vi "Heading string.vi"() -> ()   [LabVIEW 2011]
panel:
  out "String":string
  in  "Array":string[](array[string])
  out "Heading string":string
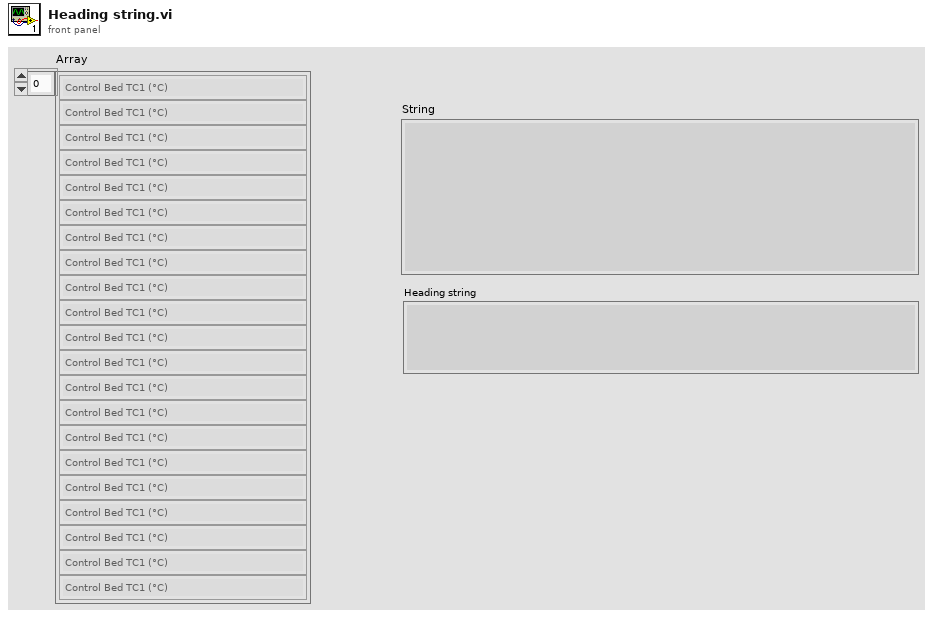
[diagram p1: front panel]
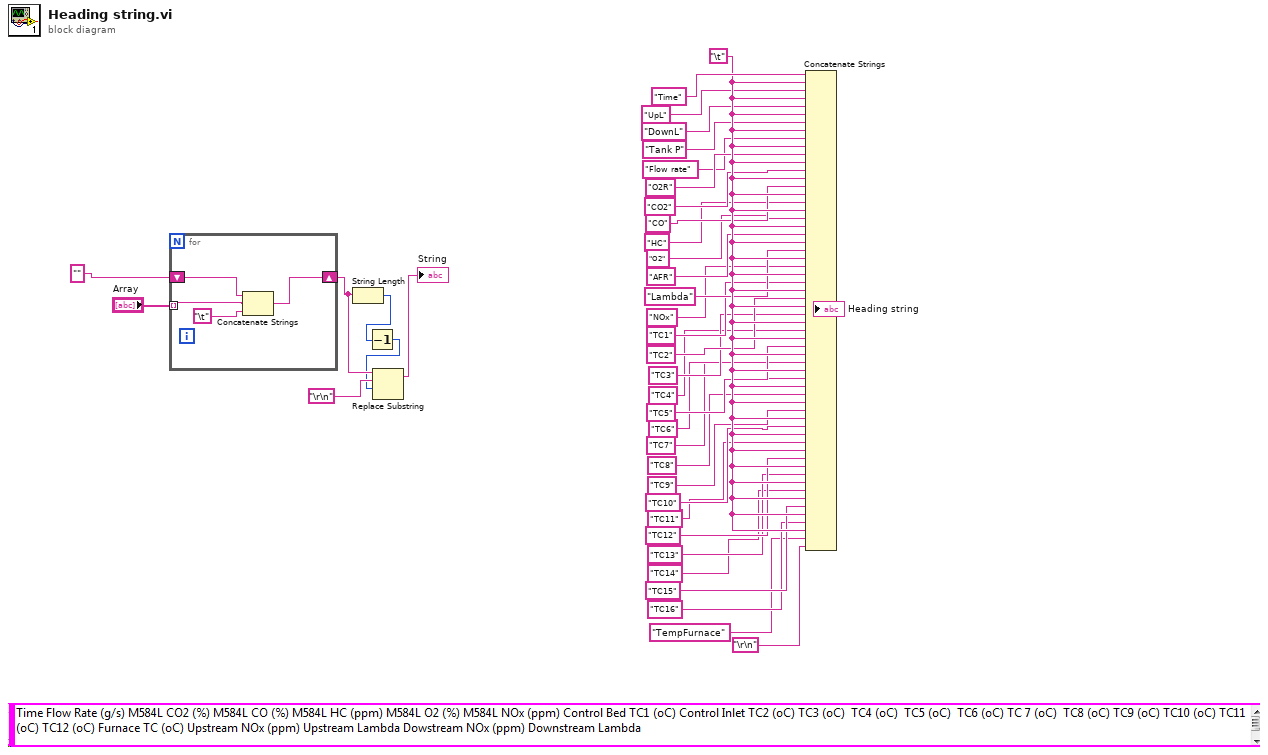
[diagram p0: block diagram]
diagram:
  w35 = "\t"
  n1 = for {
    shift-right: [w41] -> w38
    shift-left: "" -> [w42]
    tunnel: "Array" -> [w43] mode=indexing
    n2 = Concatenate Strings(w42, w43, "\t") -> (w41:string)
  }
  n3 = String Length(string=w38) -> (length=w2:i32)
  n4 = Decrement(x=w2) -> (x-1=w1:i32)
  n5 = Replace Substring(3:w1, 4:"\r\n", 5:w38) -> (1:→"String":string)  [unwired: 1 in, 1 out]
  n6 = Concatenate Strings("Time", w35, "UpL", w35, "DownL", w35, "Tank P", w35, "Flow rate", w35, "O2R", w35, "CO2", w35, "CO", w35, "HC", w35, "O2", w35, "AFR", w35, "Lambda", w35, "NOx", w35, "TC1", w35, "TC2", w35, "TC3", w35, "TC4", w35, "TC5", w35, "TC6", w35, "TC7", w35, "TC8", w35, "TC9", w35, "TC10", w35, "TC11", w35, "TC12", w35, "TC13", w35, "TC14", w35, "TC15", w35, "TC16", w35, "TempFurnace", "\r\n") -> (→"Heading string":string)
